vi "LCD.vi"(11 "String":string) -> ()   [LabVIEW 2017]
uses:
  <vilib>/myRIO/Instrument Drivers/Onboard IO/UART/typedef/VISA Configuration.ctl
  <vilib>/Instr/_visa.llb/VISA Configure Serial Port (Instr).vi
  <vilib>/myRIO/Express VI/Onboard IO/UART/UART Express VI.xnode
  <vilib>/myRIO/Instrument Drivers/Onboard IO/UART/UART.lvlib
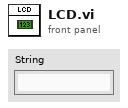
[diagram p1: front panel]
types:
  T1 = typedef "UART.lvlib/VISA Configuration.ctl" = cluster{"baud rate (9600)":u32, "data bits (8)":u16, "parity (0:none)":enum16{"None", "Odd", "Even", "Mark", "Space"}, "stop bits (10: 1 bit)":u16, "flow control (0:none)":u16, "termination char\n(0xA = '\\n' = LF) ":u8, "Enable Termination\nChar (T)":bool, "timeout (10sec)":u32}
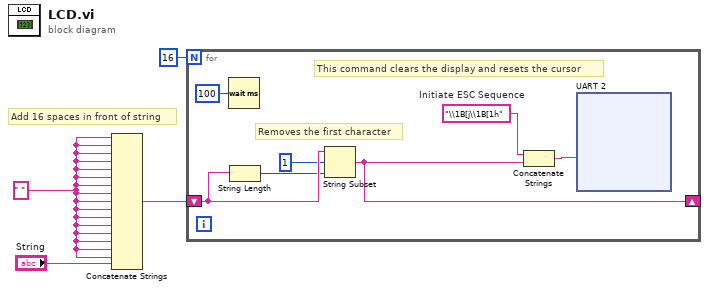
[diagram p0: block diagram]
diagram:
  w3 = " "
  # "Add 16 spaces in front of string"
  n1 = Concatenate Strings(w3, w3, w3, w3, w3, w3, w3, w3, w3, w3, w3, w3, w3, w3, w3, w3, "String") -> (w2:string)
  n2 = for {
    N: 16 -> [_]
    shift-right: [w6] -> _
    shift-left: w2 -> [w11]
    w7 = "\\1B[j\\1B[1h"  # Initiate ESC Sequence
    # "This command clears the display and resets the cursor"
    # "Removes the first character"
    n3 = Wait (ms)(milliseconds to wait=u32 100) -> ()  [unwired: 1 out]
    n4 = String Length(string=w11) -> (length=w10:i32)
    n5 = String Subset(string=w11, offset (0)=1, length (rest)=w10) -> (substring=w6:string)
    n6 = Concatenate Strings(w7, w6) -> (w5:string)
    n7 = xnode "UART 2"("Characters to Write"=w5) -> ()  [unwired: 1 in, 2 out]
  }
